vi "DelayTimer.vi"(4 "Abort Ref":refnum<vi>, 5 "Formatted \nTime Ref":refnum<vi>, 6 "FormatString":string="%M:%S", 7 "Remaining \nRef":refnum<vi>, 8 "error in (no error)":errorcluster, 11 "Delay(s)":dbl) -> (0 "error out":errorcluster)   [LabVIEW 2025]
doc: "Delay timer with formatted output available through control RefNum"
panel:
  out "FormattedTime":string
  out "remaining(s)":dbl
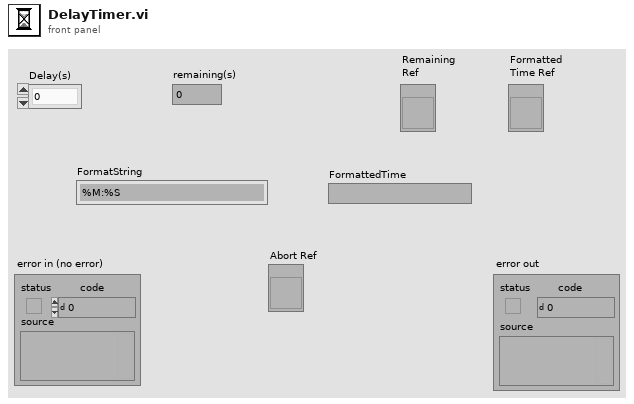
[diagram p1: front panel]
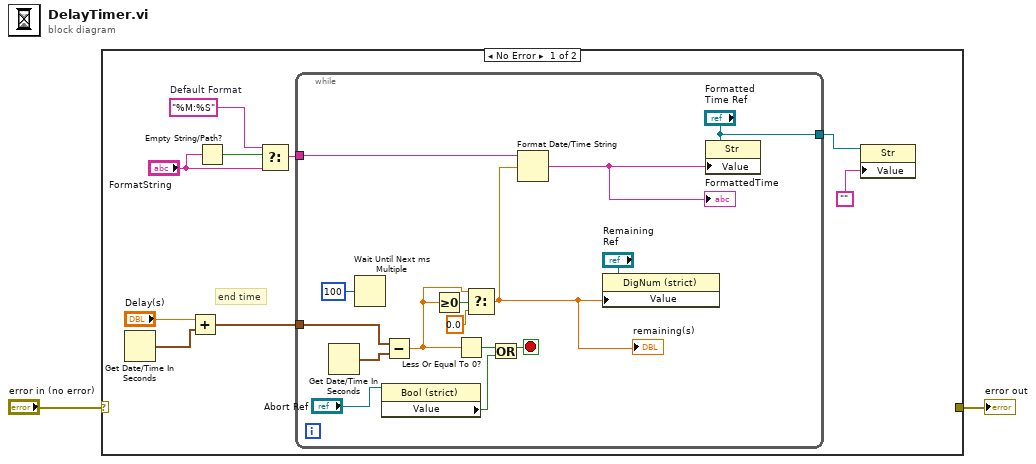
[diagram p0: block diagram]
diagram:
  n1 = case shown="No Error" "error in (no error)" {
    selector: "error in (no error)" -> [_ w27]
    tunnel: [_ w27] -> w1
    frame No Error {
      w7 = "%M:%S"  # Default Format
      # "end time"
      n2 = Get Date/Time In Seconds() -> (seconds since 1Jan1904=w10:timestamp)
      n3 = Add(x="Delay(s)", y=w10) -> (x+y=w9:timestamp)
      n4 = Empty String/Path?(string/path="FormatString") -> (empty?=w5:bool)
      n5 = Select(t=w7, s=w5, f="FormatString") -> (s? t:f=w8:string)
      n6 = while {
        tunnel: w9 -> [w25]
        tunnel: w8 -> [w22]
        tunnel: ["Formatted \nTime Ref"] -> w4
        stop <- w14 stop-if-true
        n7 = Get Date/Time In Seconds() -> (seconds since 1Jan1904=w26:timestamp)
        n8 = Wait Until Next ms Multiple(millisecond multiple=u32 100) -> ()  [unwired: 1 out]
        n9 = property class="Bool (strict)"(reference="Abort Ref") -> ("Value"=w13:bool)  [unwired: 1 in, 2 out]
        n10 = Subtract(x=w25, y=w26) -> (x-y=w19:dbl)
        n11 = Greater Or Equal To 0?(x=w19) -> (x >= 0?=w20:bool)
        n12 = Less Or Equal To 0?(x=w19) -> (x <= 0?=w24:bool)
        n13 = Select(t=w19, s=w20, f=0.0) -> (s? t:f=w18:dbl)
        "remaining(s)" <- w18
        n14 = Or(x=w24, y=w13) -> (x .or. y?=w14:bool)
        n15 = Format Date/Time String(time format string (%c)=w22, seconds (now)=w18) -> (date/time string=w17:string)  [unwired: 1 in]
        "FormattedTime" <- w17
        n16 = property class="DigNum (strict)"(reference="Remaining \nRef", "Value"=w18) -> ()  [unwired: 1 in, 2 out]
        n17 = property class="Str"(reference="Formatted \nTime Ref", "Value"=w17) -> ()  [unwired: 1 in, 2 out]
      }
      n18 = property class="Str"(reference=w4, "Value"="") -> ()  [unwired: 1 in, 2 out]
    }
    frame Error {
    }
  }
  "error out" <- w1
